vi "Track Cells.vi"(0 "Previous Image In":T1, 1 "Current Image In":T1, 3 "Process Image In":T1, 4 "Overlapped Image":T1, 5 "Objects to track In [pix]":cluster{"X":dbl, "Y":dbl}[](array[cluster]), 6 "RGB in":T1, 7 "error in":errorcluster, 8 "In":T1, 9 "Optic Flow Settings":T3={"Pyramid Levels"=6, "Max Iterations"=8, "Displacement Threshold"=0.0, "Window Size"=45}, 10 "Out":T1, 11 "Submask":T1, 12 "Window Size":cluster{"SizeX":i32, "SizeY":i32}={"SizeX"=512, "SizeY"=512}, 13 "ConvexHull":bool=TRUE, 14 "Object Type":u32(ring) items=["Bright Objects", "Dark Objects"], 15 "Track":bool, 16 "Erosion":i32(knob)=3 scale=0.0..7.0, 17 "Marker Colours":T4={"Mark (green)"=6618880, "Values (red)"=6618880, "CMs (red)"=16711680, "Rectangle (red) "=16711680}, 18 "Range Values":cluster{"Lower":dbl, "Upper":dbl}={"Lower"=1.0, "Upper"=5.0}) -> (20 "Current Image Out":T1, 21 "Overlapped Image Out":T1(plugin-control) caption="Image", 23 "All Object [pix]":T2(array[cluster]), 24 "Traced Object [pix]":T2(array[cluster]), 25 "Traced Objects CMs [pix]":cluster{"X":dbl, "Y":dbl}[](array[cluster]), 26 "RGB out":T1(plugin-control) caption="Image", 27 "error out":errorcluster)   [LabVIEW 2012, in "Visual Analyser.lvlib"]
uses:
  Visual Analyser.lvlib
  <vilib>/vision/Image Controls.llb/IMAQ Image.ctl
  <vilib>/vision/NI_Vision_Development_Module.lvlib
panel:
  in  "Number of iterations":i32=20
  out "Traced Objects Index":i32[](array[numeric])
  in  "Reject Border":bool
  out "Process":T1(plugin-control) caption="Image"
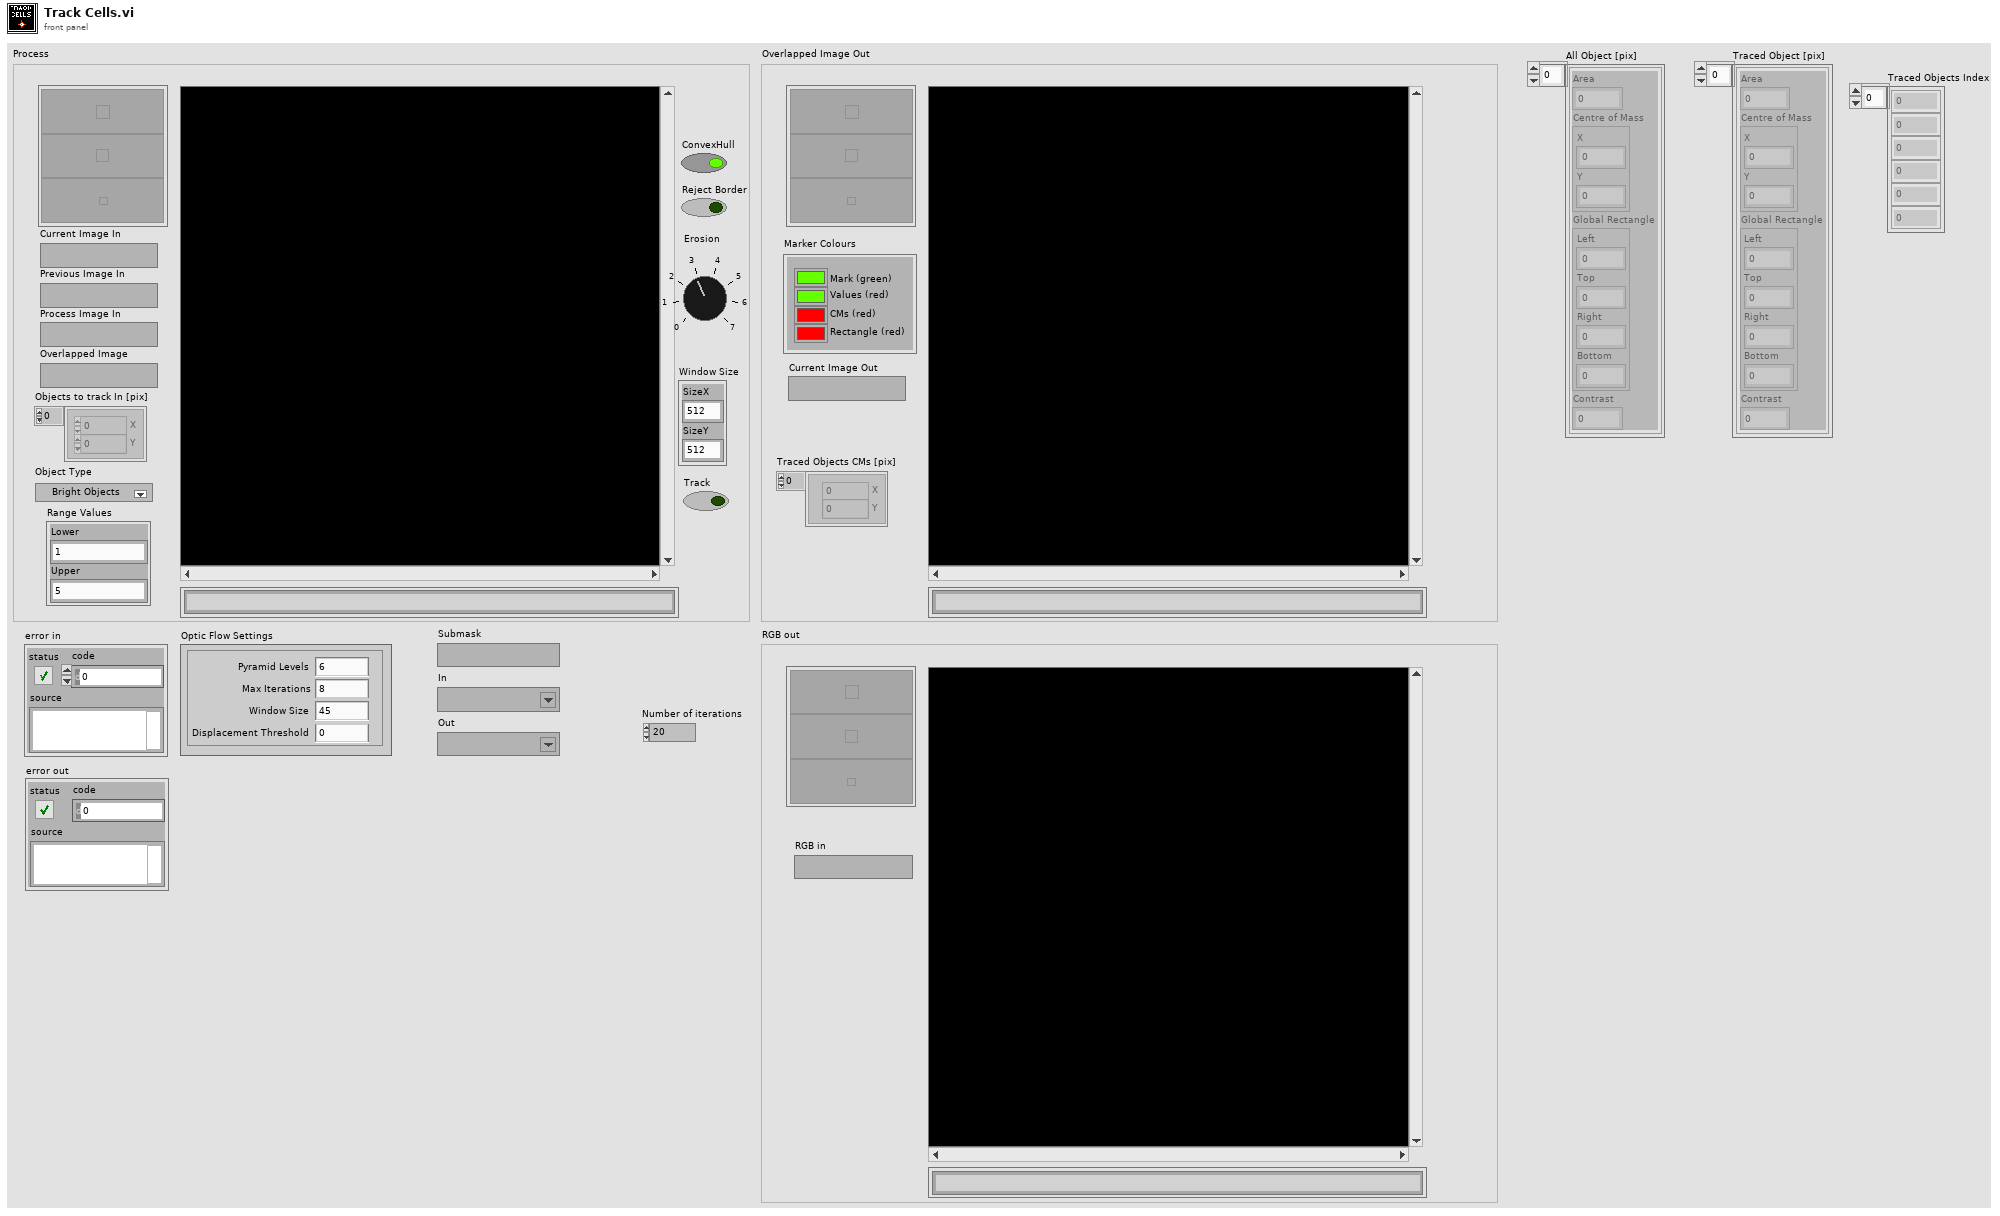
[diagram p1: front panel]
types:
  T1 = typedef "IMAQ Image.ctl" = refnum<image>
  T2 = cluster{"Area":dbl, "Centre of Mass":cluster{"X":dbl, "Y":dbl}, "Global Rectangle":cluster{"Left":dbl, "Top":dbl, "Right":dbl, "Bottom":dbl}, "Contrast":dbl}[]
  T3 = cluster{"Pyramid Levels":i32, "Max Iterations":i32, "Displacement Threshold":dbl, "Window Size":i32}
  T4 = cluster{"Mark (green)":u32, "Values (red)":u32, "CMs (red)":u32, "Rectangle (red) ":u32}
  T5 = typedef "Image Type" = u32
  T6 = typedef "Particle Parameters" = i32
  T7 = cluster{"Measurement Parameter":T6, "Range Lower Value":dbl, "Range Upper Value":dbl, "Range":bool, "Measurement Type":bool}
  T8 = cluster{"Measurement Parameter":T6, "Range Lower Value":dbl, "Range Upper Value":dbl, "Range":bool, "Measurement Type":bool}[]
  T9 = cluster{"X":dbl, "Y":dbl, "Area":dbl, "Contrast":dbl}[]
  T10 = cluster{"Left":dbl, "Top":dbl, "Right":dbl, "Bottom":dbl}[]
  T11 = cluster{"Left":dbl, "Top":dbl, "Right":dbl, "Bottom":dbl}
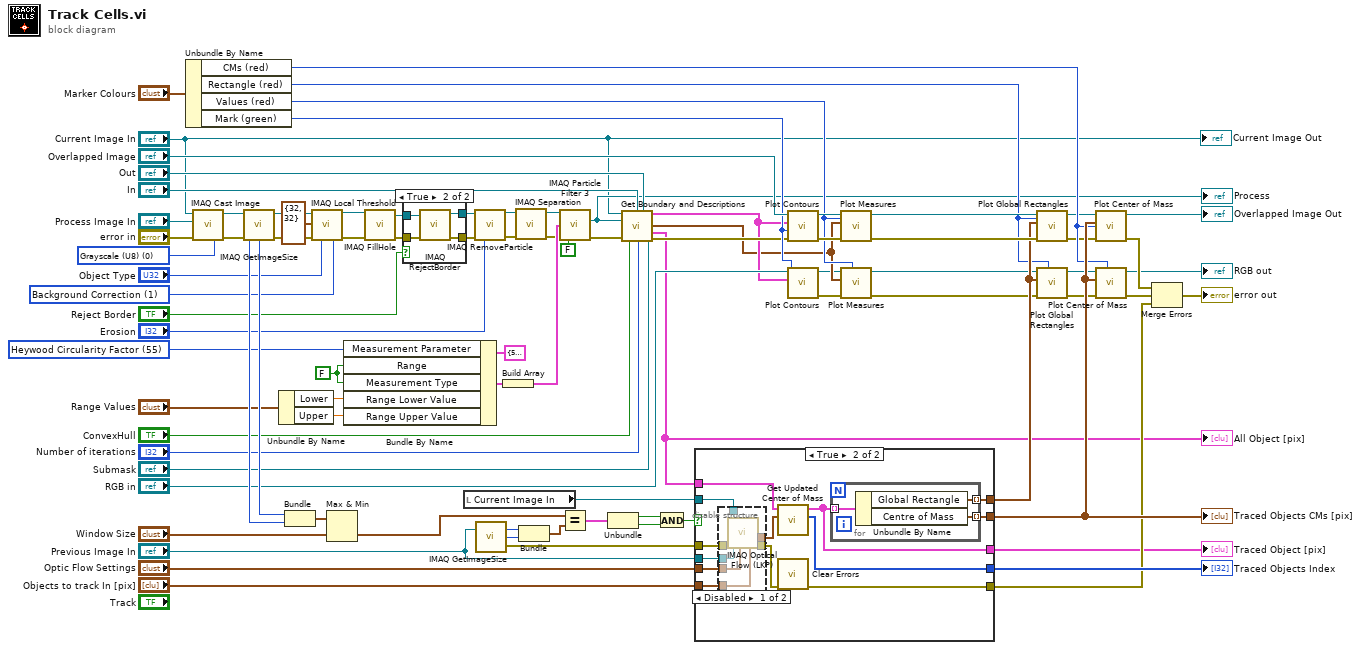
[diagram p0: block diagram]
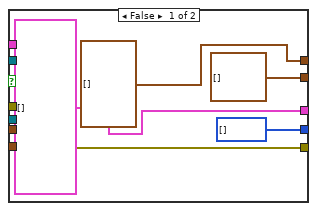
[diagram p3: hidden frame]
diagram:
  w16 = FALSE ("Keep/Remove Particles")
  w54 = T5 0 items=["Grayscale (U8)", "Grayscale (I16)", "Grayscale (SGL)", "Complex (CSG)", "RGB (U32)", "HSL (U32)", "RGB (U64)", "Grayscale (U16)"] ("Image Type")
  w75 = u32 1 items=["Niblack", "Background Correction"] ("Method (Niblack)")
  w79 = FALSE ("Range")
  w80 = T6 55 items=["Center of Mass X", "Center of Mass Y", "First Pixel X", "First Pixel Y", "Bounding Rect Left", "Bounding Rect Top", "Bounding Rect Right", "Bounding Rect Bottom", "Max Feret Diameter Start X", "Max Feret Diameter Start Y", "Max Feret Diameter End X", "Max Feret Diameter End Y", "Max Horiz. Segment Length Left", "Max Horiz. Segment Length Right", "Max Horiz. Segment Length Row", "-", "Bounding Rect Width", "Bounding Rect Height", "Bounding Rect Diagonal", "Perimeter", "Convex Hull Perimeter", "Holes' Perimeter", "Max Feret Diameter", "Equivalent Ellipse Major Axis", "Equivalent Ellipse Minor Axis", "Equivalent Ellipse Minor Axis (Feret)", "Equivalent Rect Long Side", "Equivalent Rect Short Side", "Equivalent Rect Diagonal", "Equivalent Rect Short Side (Feret)", "Average Horiz. Segment Length", "Average Vert. Segment Length", "Hydraulic Radius", "Waddel Disk Diameter", "-", "Area", "Holes' Area", "Particle & Holes' Area", "Convex Hull Area", "Image Area", "-", "Number of Holes", "Number of Horiz. Segments", "Number of Vert. Segments", "-", "Orientation", "Max Feret Diameter Orientation", "-", "% Area/Image Area", "% Area/(Particle & Holes' Area)", "Ratio of Equivalent Ellipse Axes", "Ratio of Equivalent Rect Sides", "-", "Elongation Factor", "Compactness Factor", "Heywood Circularity Factor", "Type Factor", "-", "Sum X", "Sum Y", "Sum XX", "Sum XY", "Sum YY", "Sum XXX", "Sum XXY", "Sum XYY", "Sum YYY", "-", "Moment of Inertia XX", "Moment of Inertia XY", "Moment of Inertia YY", "Moment of Inertia XXX", "Moment of Inertia XXY", "Moment of Inertia XYY", "Moment of Inertia YYY", "Norm. Moment of Inertia XX", "Norm. Moment of Inertia XY", "Norm. Moment of Inertia YY", "Norm. Moment of Inertia XXX", "Norm. Moment of Inertia XXY", "Norm. Moment of Inertia XYY", "Norm. Moment of Inertia YYY", "Hu Moment 1", "Hu Moment 2", "Hu Moment 3", "Hu Moment 4", "Hu Moment 5", "Hu Moment 6", "Hu Moment 7"] ("Measurement Parameter")
  n1 = Unbundle By Name("Marker Colours") -> ("CMs (red)"=w38:u32, "Rectangle (red)"=w37:u32, "Values (red)"=w35:u32, "Mark (green)"=w36:u32)
  n2 = call "IMAQ Cast Image"("Image Type"=w54, "error in (no error)"="error in", "Image Dst"="Process Image In", "Image Src"="Current Image In") -> ("error out"=w67:errorcluster, "Image Dst Out"=w1:T1)  [unwired: 6 in]
  n3 = call "IMAQ GetImageSize"("Image"=w1, "error in (no error)"=w67) -> ("Y Resolution"=w87:i32, "X Resolution"=w88:i32, "error out"=w76:errorcluster)  [unwired: 2 out]
  n4 = Unbundle By Name("Range Values") -> ("Lower"=w72:dbl, "Upper"=w71:dbl)
  n5 = Bundle("X Resolution"=w88, "Y Resolution"=w87) -> (w52:cluster{"X Resolution":i32, "Y Resolution":i32})  [unwired: 1 out]
  n6 = call "IMAQ Local Threshold"("Image Src"=w1, "Look For (Bright Objects)"="Object Type", "Method (Niblack)"=w75, "Window Size (32x32)"=cluster{"SizeX":i32, "SizeY":i32} {"SizeX"=32, "SizeY"=32}, "error in (no error)"=w76) -> ("Image Dst Out"=w86:T1, "error out"=w85:errorcluster)  [unwired: 3 in, 6 out]
  n7 = Max & Min(x=w52, y="Window Size") -> (min(x,y)=w60:cluster{i32, i32})  [unwired: 1 out]
  n8 = Bundle By Name(cluster=T7 {"Measurement Parameter"=55, "Range Lower Value"=0.0, "Range Upper Value"=5.0, "Range"=FALSE, "Measurement Type"=FALSE} ("Selection Value"), "Measurement Parameter"=w80, "Range"=w79, "Measurement Type"=w79, "Range Lower Value"=w72, "Range Upper Value"=w71) -> (w77:T7)
  n9 = call "IMAQ FillHole"("error in (no error)"=w85, "Image Src"=w86) -> ("error out"=w83:errorcluster, "Image Dst Out"=w84:T1)  [unwired: 2 in, 2 out]
  n10 = case shown="True" "Reject Border" {
    tunnel: w84 -> [w89 w94]
    tunnel: w83 -> [w90 w93]
    tunnel: [w89 w92] -> w82
    tunnel: [w90 w91] -> w81
    frame False {
    }
    frame True {
      n11 = call "IMAQ RejectBorder"("error in (no error)"=w93, "Image Src"=w94) -> ("error out"=w91:errorcluster, "Image Dst Out"=w92:T1)  [unwired: 2 in, 2 out]
    }
  }
  n12 = local read "Current Image In"() -> (w17:T1)
  n13 = call "IMAQ RemoveParticle"("error in (no error)"=w81, "Number of Erosion"="Erosion", "Image Src"=w82) -> ("error out"=w15:errorcluster, "Image Dst Out"=w13:T1)  [unwired: 4 in, 3 out]
  n14 = call "IMAQ GetImageSize"("Image"="Previous Image In") -> ("Y Resolution"=w63:i32, "X Resolution"=w64:i32, "error out"=w62:errorcluster)  [unwired: 3 in]
  n15 = Build Array(w77) -> (w50:T8)
  n16 = call "IMAQ Separation"("error in (no error)"=w15, "Image Src"=w13) -> ("error out"=w14:errorcluster, "Image Dst Out"=w12:T1)  [unwired: 8 in]
  n17 = Bundle("X Resolution"=w64, "Y Resolution"=w63) -> (w61:cluster{"X Resolution":i32, "Y Resolution":i32})  [unwired: 1 out]
  n18 = call "IMAQ Particle Filter 3"("Image Src"=w12, "Selection Values"=w50, "Keep/Remove Particles (F)"=w16, "error in (no error)"=w14, "Fill Holes? (F)"=w16) -> ("Image Dst Out"=w18:T1, "error out"=w19:errorcluster)  [unwired: 4 in, 5 out]
  "Process" <- w18
  n19 = Equal?(x=w60, y=w61) -> (x = y?=w59:cluster{bool, bool})
  n20 = Unbundle(w59) -> (w58:bool, w57:bool)
  n21 = call "Get Boundary and Descriptions.vi"("Image In"="Current Image In", "Number of iterations"="Number of iterations", "Out"="In", "In"="Out", "Mask In"=w18, "Submask"="Submask", "error in (no error)"=w19, "ConvexHull"="ConvexHull") -> ("Boundaries"=w28:cluster{cluster{i32, i32}[]}[], "Reporter"=w25:T9, "Object Descriptions"=w27:T2, "error out"=w32:errorcluster)  [unwired: 4 in]
  "All Object [pix]" <- w27
  n22 = And(x=w58, y=w57) -> (x .and. y?=w56:bool)
  n23 = case shown="True" w56 {
    tunnel: "Optic Flow Settings" -> [_ w102]
    tunnel: w17 -> [_ w111]
    tunnel: [w99 w100] -> w34
    tunnel: "Previous Image In" -> [_ w110]
    tunnel: w62 -> [w99 w112]
    tunnel: [T10 [] ("Enclosing Rectangles Out [pix]") w106] -> w40
    tunnel: "Objects to track In [pix]" -> [_ w109]
    tunnel: [cluster{"X":dbl, "Y":dbl}[] [] w104] -> w39
    tunnel: w27 -> [_ w107]
    tunnel: [i32[] [] ("Objects index") w105] -> w47
    tunnel: [T2 [] ("Traced Object [pix]") w103] -> w26
    frame False {
    }
    frame True {
      n24 = disable-structure shown="Disabled" {
        disable-tunnel: w112 -> [w119 w120]
        disable-tunnel: w111 -> [w118 _]
        disable-tunnel: w110 -> [w117 _]
        disable-tunnel: w109 -> [w116 w121]
        disable-tunnel: [w115 w121] -> w108
        disable-tunnel: w102 -> [w114 _]
        disable-tunnel: [w113 w120] -> w101
        frame Disabled {
          n25 = call "IMAQ Optical Flow (LKP)"("Options"=w114, "error in (no error)"=w119, "Feature Points In"=w116, "Previous Frame"=w117, "Current Frame"=w118) -> ("error out"=w113:errorcluster, "Feature Points Out"=w115:cluster{"X":sgl, "Y":sgl}[])  [unwired: 3 in, 2 out]
        }
        frame Enabled {
        }
      }
      n26 = call "Get Updated Center of Mass.vi"("Current traced points [pix]"=w108, "Objects Description[pix]"=w107) -> ("Objects index"=w105:i32[], "Traced Object [pix]"=w103:T2)  [unwired: 8 in]
      n27 = call <vilib>:"Clear Errors.vi"("error in (no error)"=w101) -> ("error out"=w100:errorcluster)  [unwired: 6 in]
      n28 = for {
        tunnel: w103 -> [w124] mode=indexing
        tunnel: [w123] -> w106 mode=indexing
        tunnel: [w122] -> w104 mode=indexing
        n29 = Unbundle By Name(w124) -> ("Global Rectangle"=w123:T11, "Centre of Mass"=w122:cluster{"X":dbl, "Y":dbl})
      }
    }
  }
  "Traced Objects CMs [pix]" <- w39
  "Traced Objects Index" <- w47
  "Traced Object [pix]" <- w26
  n30 = call "Plot Contours.vi"("error in (no error)"=w32, "Color"=w36, "Boundaries"=w28, "Image In"="Overlapped Image") -> ("error out"=w68:errorcluster, "Image"=w69:T1)  [unwired: 6 in]
  n31 = call "Plot Contours.vi"("Color"=w36, "Boundaries"=w28, "Image In"="RGB in") -> ("error out"=w7:errorcluster, "Image"=w6:T1)  [unwired: 7 in]
  n32 = call "Plot Measures.vi"("Text Color (red)"=w35, "error in"=w68, "Measurements"=w25, "Image In"=w69) -> ("error out"=w44:errorcluster, "Image Out"=w43:T1)  [unwired: 6 in]
  n33 = call "Plot Measures.vi"("Text Color (red)"=w35, "error in"=w7, "Measurements"=w25, "Image In"=w6) -> ("error out"=w10:errorcluster, "Image Out"=w11:T1)  [unwired: 6 in]
  n34 = call "Plot Global Rectangles.vi"("Text Color (red)"=w37, "error in"=w44, "Global Rectangles Array"=w40, "Image In"=w43) -> ("error out"=w4:errorcluster, "Image Out"=w5:T1)  [unwired: 6 in]
  n35 = call "Plot Global Rectangles.vi"("Text Color (red)"=w37, "error in"=w10, "Global Rectangles Array"=w40, "Image In"=w11) -> ("error out"=w9:errorcluster, "Image Out"=w8:T1)  [unwired: 6 in]
  n36 = call "Plot Center of Mass.vi"("Image"=w5, "Feature Ponts"=w39, "error in"=w4, "Color"=w38) -> ("Image Out"=→"Overlapped Image Out":T1, "error out"=w45:errorcluster)  [unwired: 5 in]
  n37 = call "Plot Center of Mass.vi"("Image"=w8, "Feature Ponts"=w39, "error in"=w9, "Color"=w38) -> ("Image Out"=→"RGB out":T1, "error out"=w33:errorcluster)  [unwired: 5 in]
  n38 = Merge Errors(w45, w33, w34) -> (→"error out":errorcluster)
  "Current Image Out" <- "Current Image In"
